vi "AddAdditionalFields.vi"(8 "error in (no error)":errorcluster, 10 "Menu":refnum<class "MGI_Menu.lvclass">, 11 "MGI_VIItem in":refnum<class "MGI_VIItem.lvclass">) -> (0 "error out":errorcluster, 2 "Menu out":refnum<class "MGI_Menu.lvclass">, 3 "MGI_VIItem out":refnum<class "MGI_VIItem.lvclass">)   [LabVIEW 2016, in "MGI_VIItem.lvclass"]
doc: "Adds shortcut hotkey to the item in the Menu\n\nAuthored by Derek E. Trepanier\nsupport@mooregoodideas.com\nwww.mooregoodideas.com\n\nCopyright (c) 2012, Moore Good Ideas, Inc.\n\nAll rights reserved.\n\nRedistribution and use in source and binary forms, with or without modification, are permitted provided that the following conditions are met:\n\n * Redistributions of source code must retain the above copyright notice, this list of conditions and the following disclaimer.\n * Redistributions in binary form must reproduce the above copyright notice, this list of conditions and the following disclaimer in the documentation and/or other materials provided with the distribution.\n * Neither the name of Moore Good Ideas, Inc. nor the names of its contributors may be used to endorse or promote products derived from this software without specific prior written permission.\n\nTHIS SOFTWARE IS PROVIDED BY THE COPYRIGHT HOLDERS AND CONTRIBUTORS \"AS IS\" AND ANY EXPRESS OR IMPLIED WARRANTIES, INCLUDING, BUT NOT LIMITED TO, THE IMPLIED WARRANTIES OF MERCHANTABILITY AND FITNESS FOR A PARTICULAR PURPOSE ARE DISCLAIMED. IN NO EVENT SHALL THE COPYRIGHT OWNER OR CONTRIBUTORS BE LIABLE FOR ANY DIRECT, INDIRECT, INCIDENTAL, SPECIAL, EXEMPLARY, OR CONSEQUENTIAL DAMAGES (INCLUDING, BUT NOT LIMITED TO, PROCUREMENT OF SUBSTITUTE GOODS OR SERVICES; LOSS OF USE, DATA, OR PROFITS; OR BUSINESS INTERRUPTION) HOWEVER CAUSED AND ON ANY THEORY OF LIABILITY, WHETHER IN CONTRACT, STRICT LIABILITY, OR TORT (INCLUDING NEGLIGENCE OR OTHERWISE) ARISING IN ANY WAY OUT OF THE USE OF THIS SOFTWARE, EVEN IF ADVISED OF THE POSSIBILITY OF SUCH DAMAGE."
uses:
  <userlib>/_MGI/Menu Building/MenuItem/VIItem/MGI_VIItem.lvclass
  C:/Program Files (x86)/National Instruments/LabVIEW 2016/user.lib/_MGI/Menu Building/MenuItem/MGI_MenuItem.lvclass
  <userlib>/_MGI/Menu Building/MenuTypes/MGI_Menu.lvclass
  <userlib>/_MGI/Menu Building/MenuTypes/Vi/MGI_VI.lvclass
  C:/Program Files (x86)/National Instruments/LabVIEW 2016/user.lib/_MGI/Menu Building/MenuTypes/MGI_Menu.lvclass
  <userlib>/_MGI/Menu Building/MenuItem/VIItem/MGI_VIItem.lvclass/MGI_VIItem.ctl
  <userlib>/_MGI/Menu Building/MenuItem/Read Tag.vi
  <userlib>/_MGI/Menu Building/MenuItem/Read Full Tag.vi
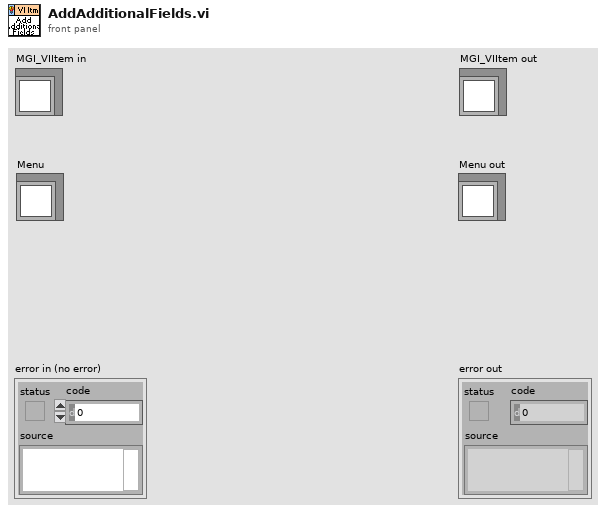
[diagram p1: front panel]
types:
  T1 = typedef "LVMenuShortCut.ctl" = cluster{"Include Shift Key?":bool, "Include Ctrl Key?":bool, "Shortcut Key":string}
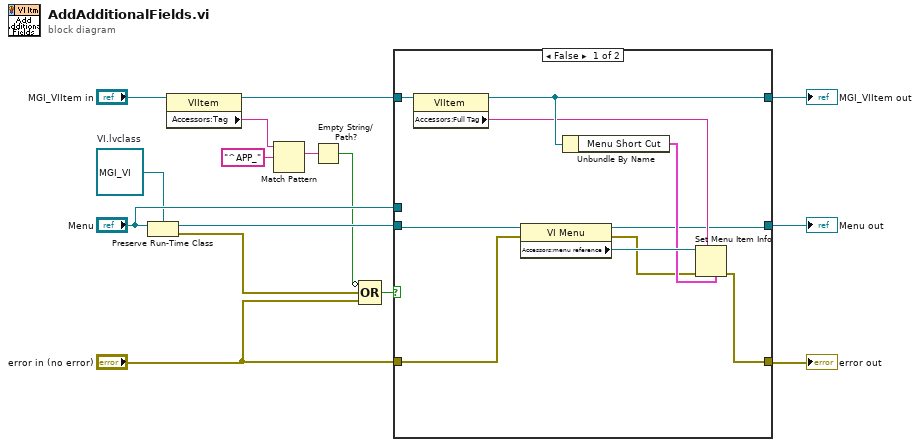
[diagram p0: block diagram]
diagram:
  w6 = refnum<class "MGI_VI.lvclass"> refnum  # VI.lvclass
  n1 = Preserve Run-Time Class(object in="Menu", 2:w6) -> (object out=w11:refnum<class "MGI_VI.lvclass">, error out=w8:errorcluster)  [unwired: 1 in]
  n2 = property class="VIItem"(reference="MGI_VIItem in") -> (reference out=w3:refnum<class "MGI_VIItem.lvclass">, "Accessors:Tag"=w2:string)  [unwired: 1 in, 1 out]
  n3 = Match Pattern(string=w2, regular expression="^APP_") -> (match substring=w4:string)  [unwired: 1 in, 3 out]
  n4 = Empty String/Path?(string/path=w4) -> (empty?=w1:bool)
  n5 = Compound Arithmetic op=OR(invert w1, w8, "error in (no error)") -> (w9:bool)
  n6 = case shown="False" w9 {
    tunnel: [w17 w26] -> w15
    tunnel: [w21 w28] -> w14
    tunnel: w3 -> [w22 w28]
    tunnel: [w19 w27] -> w12
    tunnel: w11 -> [w25 _]
    tunnel: "Menu" -> [_ w27]
    tunnel: "error in (no error)" -> [w16 w26]
    frame False {
      n7 = property class="VIItem"(reference=w22) -> (reference out=w21:refnum<class "MGI_VIItem.lvclass">, "Accessors:Full Tag"=w20:string)  [unwired: 1 in, 1 out]
      n8 = property class="VI Menu"(reference=w25, error in=w16) -> (reference out=w19:refnum<class "MGI_VI.lvclass">, error out=w18:errorcluster, "Accessors:menu reference"=w24:refnum<k9>)
      n9 = Unbundle By Name(w21) -> ("Menu Short Cut"=w23:T1)
      n10 = Set Menu Item Info(4:w23, 7:w20, 8:w18, 11:w24) -> (0:w17:errorcluster)  [unwired: 3 in, 1 out]
    }
    frame True {
      # "I dont want the cast error to propogate, but i do want it\nto cause a no-op"
    }
  }
  "error out" <- w15
  "MGI_VIItem out" <- w14
  "Menu out" <- w12
